vi "Autonomous_Parse.vi"(0 "File Path":path=path "C:/Users/theST/Desktop/Autonomous/Test.txt", 11 "error in":errorcluster) -> (1 "Name of Play":string, 3 "DS Message":string, 4 "Number of Commands":i32, 6 "Subsystems":string[](array[string]), 8 "Commands":string[](array[string]), 10 "Inputs":string[][](array[string]), 15 "errror out":errorcluster)   [LabVIEW 2019]
uses:
  <vilib>/Utility/file.llb/Read Delimited Spreadsheet (string).vi
panel:
  out "Lines":string[](array[string])
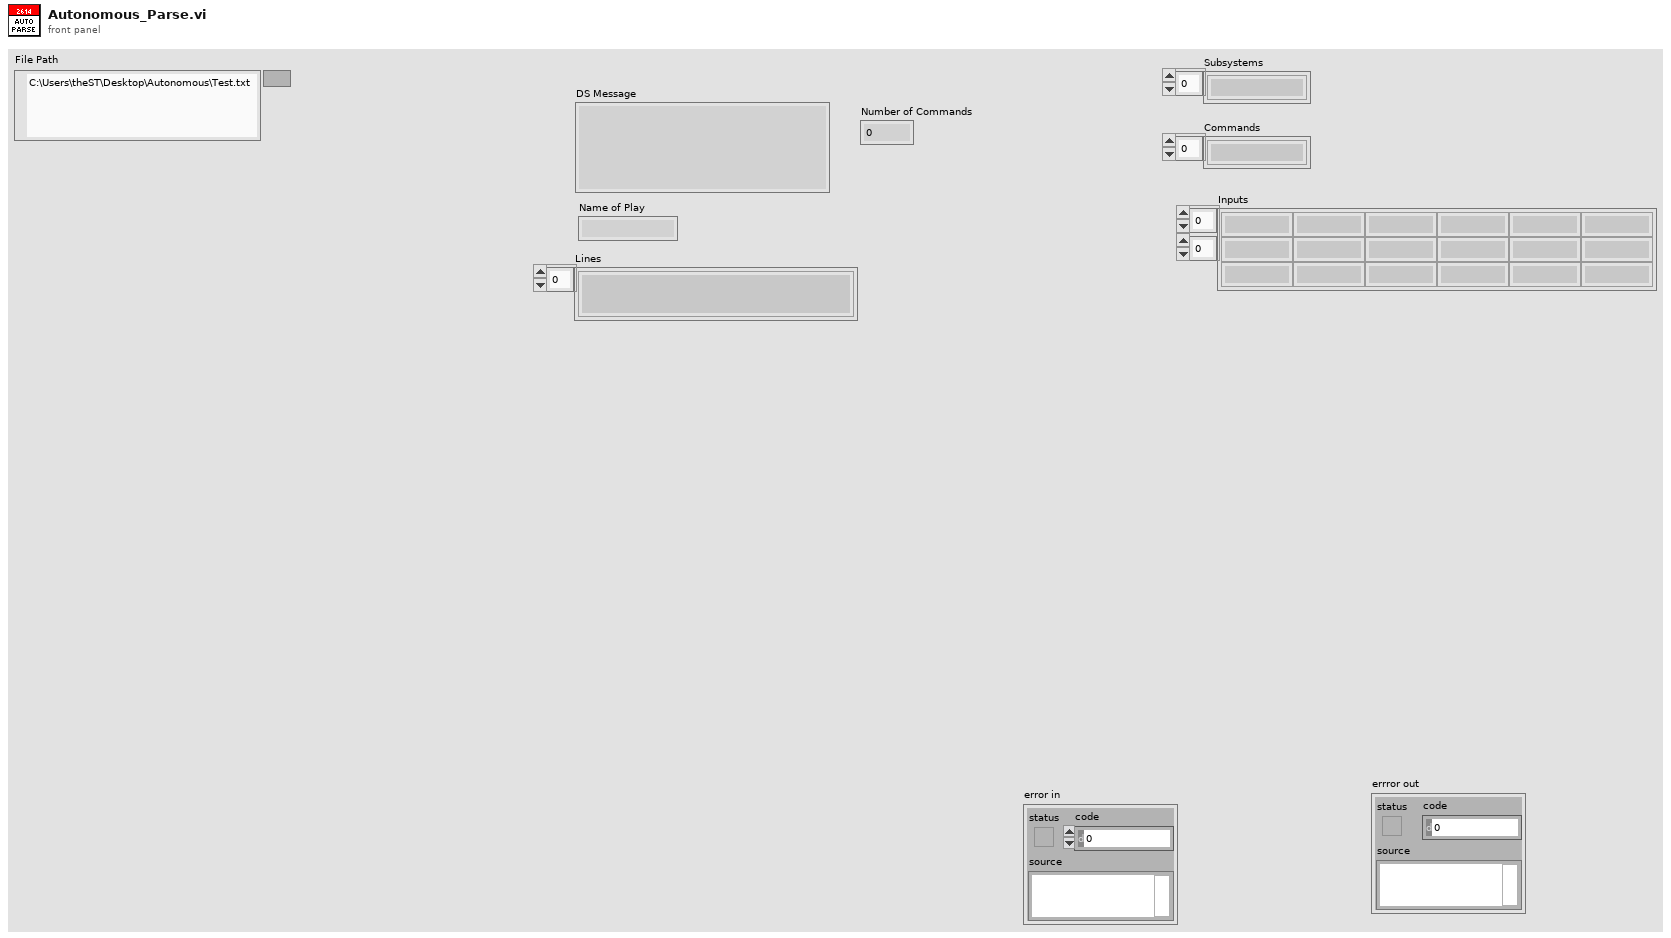
[diagram p1: front panel]
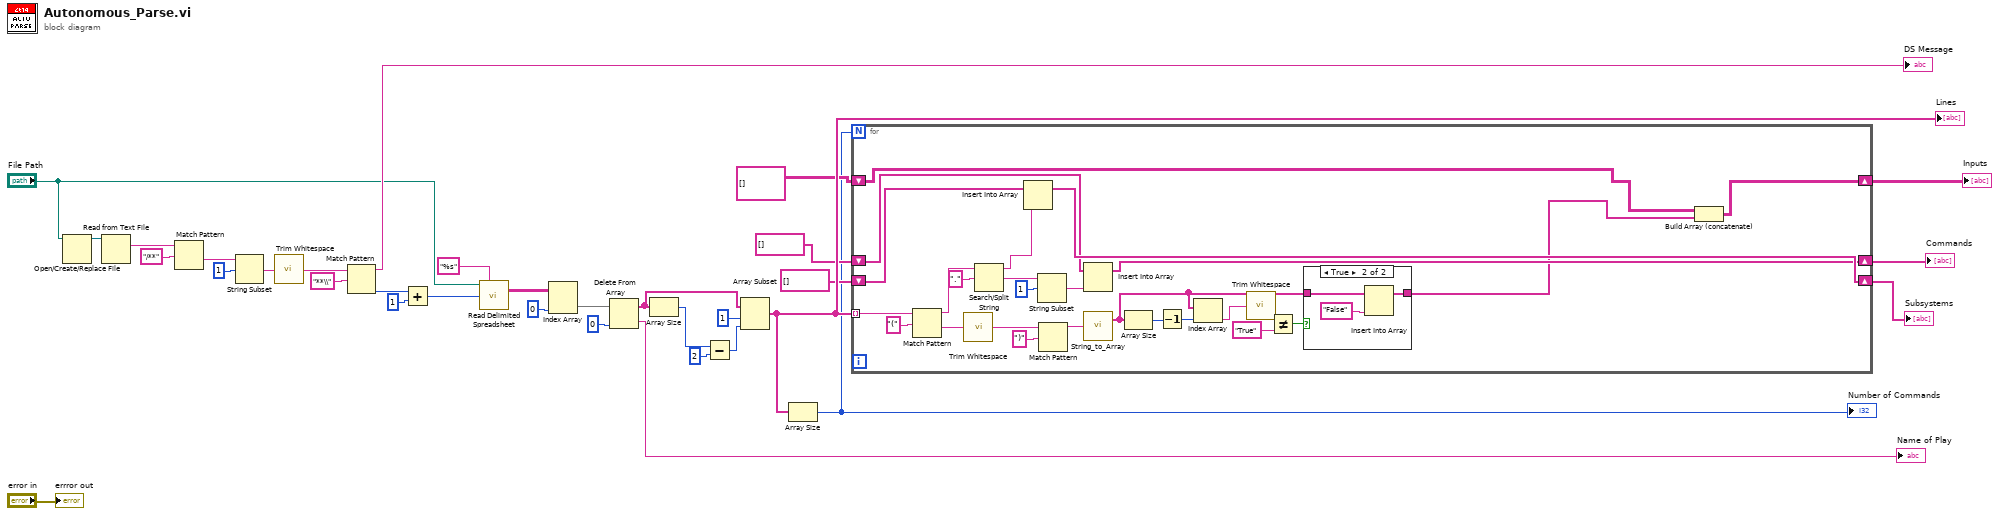
[diagram p0: block diagram]
diagram:
  n1 = Open/Create/Replace File(file path (use dialog)="File Path") -> (refnum out=w33:refnum<file>)  [unwired: 5 in, 2 out]
  n2 = Read from Text File(file (use dialog)=w33) -> (text=w8:string)  [unwired: 3 in, 3 out]
  n3 = Match Pattern(string=w8, regular expression="/**") -> (after substring=w31:string)  [unwired: 1 in, 3 out]
  n4 = String Subset(string=w31, offset (0)=1) -> (substring=w27:string)  [unwired: 1 in]
  n5 = call <vilib>:"Trim Whitespace.vi"("string"=w27) -> ("trimmed string"=w26:string)  [unwired: 1 in]
  n6 = Match Pattern(string=w26, regular expression="**\\") -> (before substring=→"DS Message":string, offset past match=w14:i32)  [unwired: 1 in, 2 out]
  n7 = Add(x=w14, y=1) -> (x+y=w13:i32)
  n8 = call-poly <vilib>:"Read Delimited Spreadsheet.vi"("file path (dialog if empty)"="File Path", "format (%s)"="%s", "start of read offset (chars.:0)"=w13) -> ("all rows"=w16:string[][])  [unwired: 7 in, 5 out]
  n9 = Index Array(array=w16, index (col)=0 ("disabled index (col)")) -> (element=w20:string[])  [unwired: 1 in]
  n10 = Delete From Array(array=w20, index=0) -> (deleted portion=→"Name of Play":string, array with subset deleted=w21:string[])  [unwired: 1 in]
  n11 = Array Size(array=w21) -> (size(s)=w24:i32)
  n12 = Subtract(x=w24, y=2) -> (x-y=w23:i32)
  n13 = Array Subset(array=w21, index=1, length=w23) -> (w11:string[])
  "Lines" <- w11
  n14 = Array Size(array=w11) -> (size(s)=w2:i32)
  "Number of Commands" <- w2
  n15 = for {
    N: w2 -> [_]
    tunnel: w11 -> [w56] mode=indexing
    shift-right: [w38] -> w1
    shift-left: string[][] [] ("appended array") -> [w40]
    shift-right: [w53] -> w10
    shift-left: string[] [] -> [w51]
    shift-right: [w52] -> w3
    shift-left: string[] [] -> [w50]
    n16 = Match Pattern(string=w56, regular expression="(") -> (before substring=w48:string, after substring=w59:string)  [unwired: 1 in, 2 out]
    n17 = call <vilib>:"Trim Whitespace.vi"("string"=w59) -> ("trimmed string"=w57:string)  [unwired: 1 in]
    n18 = Search/Split String(string=w48, search string/char (-)=".") -> (substring before match=w47:string, match + rest of string=w45:string)  [unwired: 1 in, 1 out]
    n19 = Insert Into Array(array=w51, new element=w47) -> (w53:string[])  [unwired: 1 in]
    n20 = String Subset(string=w45, offset (0)=1) -> (substring=w37:string)  [unwired: 1 in]
    n21 = Match Pattern(string=w57, regular expression=")") -> (before substring=w54:string)  [unwired: 1 in, 3 out]
    n22 = Insert Into Array(array=w50, new element=w37) -> (w52:string[])  [unwired: 1 in]
    n23 = call "String_to_Array.vi"("Input String"=w54) -> ("Array of Strings"=w42:string[])  [unwired: 1 out]
    n24 = Array Size(array=w42) -> (size(s)=w44:i32)
    n25 = Decrement(x=w44) -> (x-1=w43:i32)
    n26 = Index Array(array=w42, index=w43) -> (element=w35:string)
    n27 = call <vilib>:"Trim Whitespace.vi"("string"=w35) -> ("trimmed string"=w34:string)  [unwired: 1 in]
    n28 = Not Equal?(x=w34, y="True") -> (x != y?=w41:bool)
    n29 = case shown="True" w41 {
      tunnel: w42 -> [w60 w63]
      tunnel: [w60 w61] -> w39
      frame False {
      }
      frame True {
        n30 = Insert Into Array(array=w63, new element="False" ("new element/subarray")) -> (w61:string[])  [unwired: 1 in]
      }
    }
    n31 = Build Array (concatenate)(w40, w39) -> (w38:string[][])
  }
  "Subsystems" <- w10
  "Inputs" <- w1
  "Commands" <- w3
  "errror out" <- "error in"
